vi "Sample CORE Mssg (BORRAR).vi"() -> ()   [LabVIEW 2014]
panel:
  out "DO 5":bool[](array[boolean])
  out "DO 4":bool[](array[boolean])
  out "DO 3":bool[](array[boolean])
  out "DO 2":bool[](array[boolean])
  out "HWAsync 10":string
  out "HWAsync 9":string
  out "HWAsync 8":string
  out "HWAsync 7":string
  out "HWAsync 6":string
  out "HWAsync 5":string
  out "HWAsync 4":string
  out "HWAsync 3":string
  out "HWAsync 2":string
  out "HWSync 5":string
  out "HWSync 4":string
  out "HWSync 3":string
  out "HWSync 2":string
  out "MATH":string
  out "DO 1":bool[](array[boolean])
  out "HWAsync 1":string
  out "HWSync 1":string
  # "Dispositivos SINCRONOS"
  # "Dispositivos ASINCRONOS"
  # "Módulo MATEMATICO"
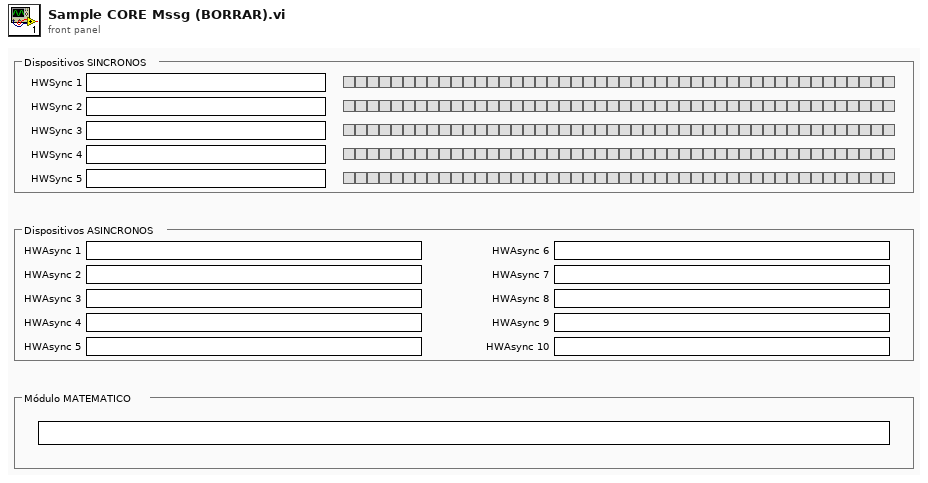
[diagram p1: front panel]
types:
  T1 = cluster{"format string":string, "Measurement Index":i32[]}
  T2 = cluster{"MAX(T) or MIN (F)?":bool, "Mastering TDX Index":i32[]}
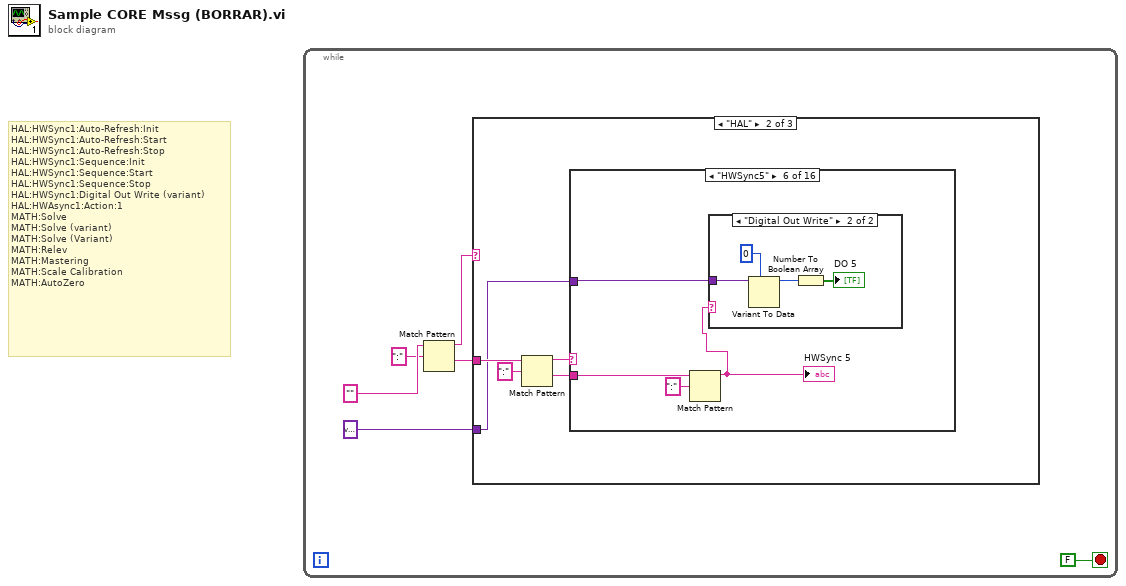
[diagram p0: block diagram]
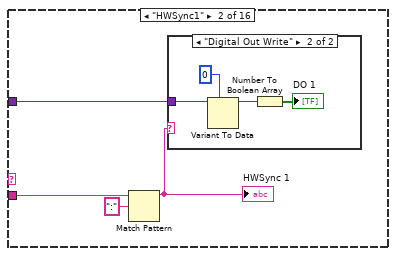
[diagram p4: hidden frame]
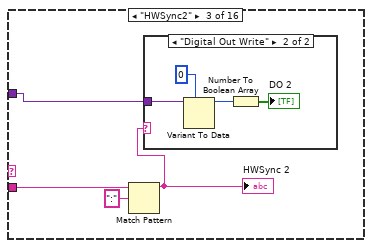
[diagram p6: hidden frame]
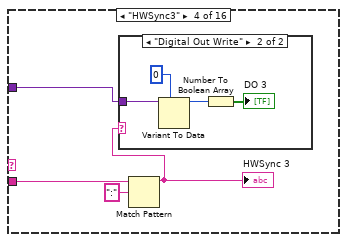
[diagram p8: hidden frame]
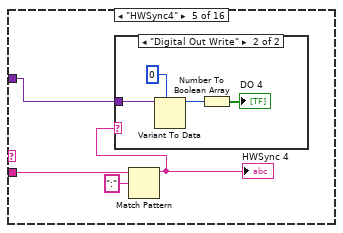
[diagram p10: hidden frame]
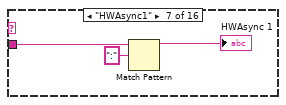
[diagram p13: hidden frame]
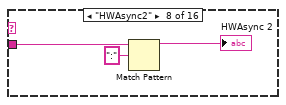
[diagram p14: hidden frame]
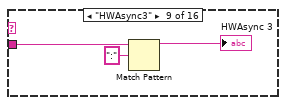
[diagram p15: hidden frame]
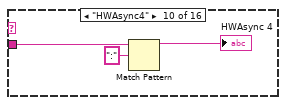
[diagram p16: hidden frame]
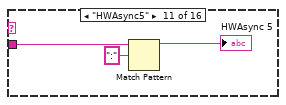
[diagram p17: hidden frame]
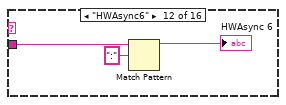
[diagram p18: hidden frame]
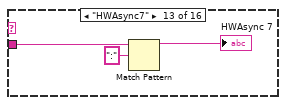
[diagram p19: hidden frame]
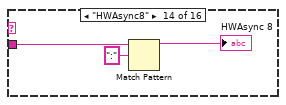
[diagram p20: hidden frame]
diagram:
  # "HAL:HWSync1:Auto-Refresh:Init\nHAL:HWSync1:Auto-Refresh:Start\nHAL:HWSync1:Auto-Refresh:Stop\nHAL:HWSync1:Sequence:Init\nHAL:HWSync1:Sequence:Start\nHAL:HWSync1:Sequence:Stop\nHAL:HWSync1:Digital Out Write (variant)\nHAL:HWAsync1:Action:1\nMATH:Solve\nMATH:Solve (variant)\nMATH:Solve (Variant)\nMATH:Relev\nMATH:Mastering\nMATH:Scale Calibration\nMATH:AutoZero"
  n1 = while {
    stop <- FALSE stop-if-true
    n2 = Match Pattern(string="" ("String"), regular expression=":") -> (before substring=w4:string, after substring=w3:string)  [unwired: 1 in, 2 out]
    n3 = case shown="\"HAL\"" w4 {
      tunnel: w3 -> [_ w10 w83]
      tunnel: variant -> [_ w7 w84]
      frame Default {
      }
      frame "HAL" {
        n4 = Match Pattern(string=w10, regular expression=":") -> (before substring=w9:string, after substring=w8:string)  [unwired: 1 in, 2 out]
        n5 = case shown="\"HWSync5\"" w9 {
          tunnel: w8 -> [_ w14 w22 w30 w38 w46 w53 w56 w59 w62 w65 w68 w71 w74 w77 w80]
          tunnel: w7 -> [_ w13 w20 w29 w37 w45 _ _ _ _ _ _ _ _ _ _]
          frame "False", Default {
          }
          frame "HWSync1" {
            n6 = Match Pattern(string=w14, regular expression=":") -> (before substring=w12:string)  [unwired: 1 in, 3 out]
            "HWSync 1" <- w12
            n7 = case shown="\"Digital Out Write\"" w12 {
              tunnel: w13 -> [_ w19]
              frame "False", Default {
              }
              frame "Digital Out Write" {
                n8 = Variant To Data(type=0, Variant=w19) -> (data=w17:i32)  [unwired: 1 in, 1 out]
                n9 = Number To Boolean Array(number=w17) -> (Boolean array=→"DO 1":bool[])
              }
            }
          }
          frame "HWSync2" {
            n10 = Match Pattern(string=w22, regular expression=":") -> (before substring=w21:string)  [unwired: 1 in, 3 out]
            "HWSync 2" <- w21
            n11 = case shown="\"Digital Out Write\"" w21 {
              tunnel: w20 -> [_ w27]
              frame "False", Default {
              }
              frame "Digital Out Write" {
                n12 = Variant To Data(type=0, Variant=w27) -> (data=w25:i32)  [unwired: 1 in, 1 out]
                n13 = Number To Boolean Array(number=w25) -> (Boolean array=→"DO 2":bool[])
              }
            }
          }
          frame "HWSync3" {
            n14 = Match Pattern(string=w30, regular expression=":") -> (before substring=w28:string)  [unwired: 1 in, 3 out]
            "HWSync 3" <- w28
            n15 = case shown="\"Digital Out Write\"" w28 {
              tunnel: w29 -> [_ w35]
              frame "False", Default {
              }
              frame "Digital Out Write" {
                n16 = Variant To Data(type=0, Variant=w35) -> (data=w33:i32)  [unwired: 1 in, 1 out]
                n17 = Number To Boolean Array(number=w33) -> (Boolean array=→"DO 3":bool[])
              }
            }
          }
          frame "HWSync4" {
            n18 = Match Pattern(string=w38, regular expression=":") -> (before substring=w36:string)  [unwired: 1 in, 3 out]
            "HWSync 4" <- w36
            n19 = case shown="\"Digital Out Write\"" w36 {
              tunnel: w37 -> [_ w43]
              frame "False", Default {
              }
              frame "Digital Out Write" {
                n20 = Variant To Data(type=0, Variant=w43) -> (data=w41:i32)  [unwired: 1 in, 1 out]
                n21 = Number To Boolean Array(number=w41) -> (Boolean array=→"DO 4":bool[])
              }
            }
          }
          frame "HWSync5" {
            n22 = Match Pattern(string=w46, regular expression=":") -> (before substring=w44:string)  [unwired: 1 in, 3 out]
            "HWSync 5" <- w44
            n23 = case shown="\"Digital Out Write\"" w44 {
              tunnel: w45 -> [_ w51]
              frame "False", Default {
              }
              frame "Digital Out Write" {
                n24 = Variant To Data(type=0, Variant=w51) -> (data=w49:i32)  [unwired: 1 in, 1 out]
                n25 = Number To Boolean Array(number=w49) -> (Boolean array=→"DO 5":bool[])
              }
            }
          }
          frame "HWAsync1" {
            n26 = Match Pattern(string=w53, regular expression=":") -> (before substring=→"HWAsync 1":string)  [unwired: 1 in, 3 out]
          }
          frame "HWAsync2" {
            n27 = Match Pattern(string=w56, regular expression=":") -> (before substring=→"HWAsync 2":string)  [unwired: 1 in, 3 out]
          }
          frame "HWAsync3" {
            n28 = Match Pattern(string=w59, regular expression=":") -> (before substring=→"HWAsync 3":string)  [unwired: 1 in, 3 out]
          }
          frame "HWAsync4" {
            n29 = Match Pattern(string=w62, regular expression=":") -> (before substring=→"HWAsync 4":string)  [unwired: 1 in, 3 out]
          }
          frame "HWAsync5" {
            n30 = Match Pattern(string=w65, regular expression=":") -> (before substring=→"HWAsync 5":string)  [unwired: 1 in, 3 out]
          }
          frame "HWAsync6" {
            n31 = Match Pattern(string=w68, regular expression=":") -> (before substring=→"HWAsync 6":string)  [unwired: 1 in, 3 out]
          }
          frame "HWAsync7" {
            n32 = Match Pattern(string=w71, regular expression=":") -> (before substring=→"HWAsync 7":string)  [unwired: 1 in, 3 out]
          }
          frame "HWAsync8" {
            n33 = Match Pattern(string=w74, regular expression=":") -> (before substring=→"HWAsync 8":string)  [unwired: 1 in, 3 out]
          }
          frame "HWAsync9" {
            n34 = Match Pattern(string=w77, regular expression=":") -> (before substring=→"HWAsync 9":string)  [unwired: 1 in, 3 out]
          }
          frame "HWAsync10" {
            n35 = Match Pattern(string=w80, regular expression=":") -> (before substring=→"HWAsync 10":string)  [unwired: 1 in, 3 out]
          }
        }
      }
      frame "MATH" {
        n36 = case shown="\"Solve\"" w83 {
          tunnel: w84 -> [_ w91 w143 w157 w167 _]
          tunnel: ["" ("format string") w86 w140 w156 w164 "Calcular Constantes de calibracion de Balanzas" ("format string")] -> w82
          frame Default {
          }
          frame "Solve" {
            n37 = Variant To Data(type=T1 {"format string"="", "Measurement Index"=[]} ("output cluster"), Variant=w91) -> (data=w89:T1)  [unwired: 1 in, 1 out]
            n38 = Unbundle(w89) -> ("format string"=w88:string, "Measurement Index"=w87:i32[])
            n39 = case shown="\"Relev\"" w88 {
              tunnel: w87 -> [_ w99 w111 w123]
              tunnel: ["-" w93 w105 w117] -> w86
              frame Default {
              }
              frame "\u0000" {
                n40 = Number To Decimal String(number=w99) -> (decimal integer string=w98:string[])  [unwired: 1 in]
                n41 = for {
                  tunnel: w98 -> [w103] mode=indexing
                  shift-right: [w104] -> w96
                  shift-left: "[ " ("String") -> [w100]
                  n42 = Concatenate Strings(w100, "M" ("string"), w103, " " ("String")) -> (w104:string)
                }
                n43 = Concatenate Strings("Resolver Mediciones -> " ("format string"), w96, "]" ("String")) -> (w93:string)
              }
              frame "Relev" {
                n44 = Number To Decimal String(number=w111) -> (decimal integer string=w110:string[])  [unwired: 1 in]
                n45 = for {
                  tunnel: w110 -> [w115] mode=indexing
                  shift-right: [w116] -> w108
                  shift-left: "[ " ("String") -> [w112]
                  n46 = Concatenate Strings(w112, "M" ("string"), w115, " " ("String")) -> (w116:string)
                }
                n47 = Concatenate Strings("Resolver Mediciones con relevamiento de Pieza Patron -> " ("format string"), w108, "]" ("String")) -> (w105:string)
              }
              frame "Mastering" {
                n48 = Number To Decimal String(number=w123) -> (decimal integer string=w122:string[])  [unwired: 1 in]
                n49 = for {
                  tunnel: w122 -> [w127] mode=indexing
                  shift-right: [w128] -> w120
                  shift-left: "[ " ("String") -> [w124]
                  n50 = Concatenate Strings(w124, "M" ("string"), w127, " " ("String")) -> (w128:string)
                }
                n51 = Concatenate Strings("Resolver Mediciones con Mastering -> " ("format string"), w120, "]" ("String")) -> (w117:string)
              }
            }
          }
          frame "Mastering" {
            n52 = Variant To Data(type=T2 {"MAX(T) or MIN (F)?"=FALSE, "Mastering TDX Index"=[]} ("output cluster"), Variant=w143) -> (data=w142:T2)  [unwired: 1 in, 1 out]
            n53 = Unbundle(w142) -> ("MAX(T) or MIN (F)?"=w134:bool, "Mastering TDX Index"=w141:i32[])
            n54 = Number To Decimal String(number=w141) -> (decimal integer string=w139:string[])  [unwired: 1 in]
            n55 = Select(t="MAXIMO" ("format string"), s=w134, f="MINIMO" ("format string")) -> (s? t:f=w130:string)
            n56 = for {
              tunnel: w139 -> [w147] mode=indexing
              shift-right: [w148] -> w137
              shift-left: "[ " ("String") -> [w144]
              n57 = Concatenate Strings(w144, "T" ("string"), w147, " " ("String")) -> (w148:string)
            }
            n58 = Format Into String(format string="Tomar %s de los Transductores ->", w130) -> (resulting string=w129:string)  [unwired: 2 in, 1 out]
            n59 = Concatenate Strings(w129, w137, "]" ("String")) -> (w140:string)
          }
          frame "AutoZero" {
            n60 = Variant To Data(type=i32[] [] ("Mastering TDX Index"), Variant=w157) -> (data=w149:i32[])  [unwired: 1 in, 1 out]
            n61 = Number To Decimal String(number=w149) -> (decimal integer string=w155:string[])  [unwired: 1 in]
            n62 = for {
              tunnel: w155 -> [w161] mode=indexing
              shift-right: [w162] -> w153
              shift-left: "[ " ("String") -> [w158]
              n63 = Concatenate Strings(w158, "T" ("string"), w161, " " ("String")) -> (w162:string)
            }
            n64 = Concatenate Strings("Calcular Zero de los Transductores ->" ("format string"), w153, "]" ("String")) -> (w156:string)
          }
          frame "Relev" {
            n65 = Variant To Data(type=0, Variant=w167) -> (data=w163:i32)  [unwired: 1 in, 1 out]
            n66 = Format Into String(format string="Calcular Relevamiento de Pieza Patron en Transductor T%d", w163) -> (resulting string=w164:string)  [unwired: 2 in, 1 out]
          }
          frame "Scale Calibrate" {
          }
        }
        "MATH" <- w82
      }
    }
  }
